vi "VI Tree.vi"   [LabVIEW 2012, in "Phidget Power Guard.lvlib"]
doc: "${PowerGuard:VITreeHeader}"
uses:
  <instrlib>/Phidgets/Phidget Power Guard/Phidget Power Guard.lvlib
  <instrlib>/Phidgets/Phidget Power Guard/Public/PowerGuardStart.vi
  <instrlib>/Phidgets/Phidget Power Guard/Public/PowerGuardOpen.vi
  <instrlib>/Phidgets/Phidget Power Guard/Public/PowerGuardClose.vi
  <instrlib>/Phidgets/Phidget Common/Phidget Common.lvlib
panel:
  # "(c) 2015 Phidgets Inc..  ALL RIGHTS RESERVED."
  # "SEE DIAGRAM\nFOR VI TREE."
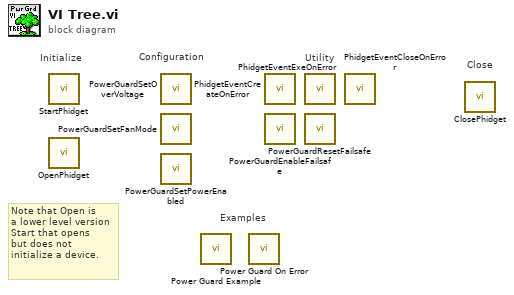
[diagram p0: block diagram]
diagram:
  # "Note that Open is\na lower level version\nStart that opens\nbut does not \ninitialize a device."
  # "Examples"
  # "Configuration"
  # "Utility"
  # "Close"
  # "Initialize"
  n1 = call-poly <instrlib>:"StartPhidget.vi"() -> ()  [unwired: 12 in, 4 out]
  n2 = call-poly <instrlib>:"OpenPhidget.vi"() -> ()  [unwired: 8 in, 4 out]
  n3 = call <instrlib>:"PowerGuardSetOverVoltage.vi"() -> ()  [unwired: 9 in, 2 out]
  n4 = call <instrlib>:"PowerGuardSetFanMode.vi"() -> ()  [unwired: 9 in, 2 out]
  n5 = call <instrlib>:"PowerGuardSetPowerEnabled.vi"() -> ()  [unwired: 9 in, 2 out]
  n6 = call <instrlib>:"Power Guard Example.vi"() -> ()  [unwired: 12 in]
  n7 = call <instrlib>:"Power Guard On Error.vi"() -> ()  [unwired: 12 in]
  n8 = call <instrlib>:"PhidgetEventCreateOnError.vi"() -> ()  [unwired: 9 in, 3 out]
  n9 = call <instrlib>:"PowerGuardEnableFailsafe.vi"() -> ()  [unwired: 9 in, 2 out]
  n10 = call <instrlib>:"PhidgetEventExeOnError.vi"() -> ()  [unwired: 8 in, 8 out]
  n11 = call <instrlib>:"PowerGuardResetFailsafe.vi"() -> ()  [unwired: 9 in, 2 out]
  n12 = call <instrlib>:"PhidgetEventCloseOnError.vi"() -> ()  [unwired: 10 in, 2 out]
  n13 = call-poly <instrlib>:"ClosePhidget.vi"() -> ()  [unwired: 11 in, 1 out]
